vi "test Loopback_Complex_withOverflow.vi"(8 "error in":errorcluster, 11 "TestCase in":refnum<class "Single Core Complex Loopback.lvclass">) -> (0 "error out":errorcluster, 3 "TestCase out":refnum<class "Single Core Complex Loopback.lvclass">)   [LabVIEW 2020, in "Single Core Complex Loopback.lvclass"]
uses:
  Single Core Complex Loopback.lvclass
  <vilib>/addons/_JKI Toolkits/VI Tester/TestCase.llb/TestCase.lvclass
  4b06c685-66bb-4135-9ad1-d89a50a95502.vi
  <vilib>/NI VeriStand/Execution/Workspace/NI_VS Workspace ExecutionAPI.lvlib
  <vilib>/NI VeriStand/Execution/Workspace/NI VeriStand - Get Single Channel Value.vi
  <vilib>/numeric/Random Number (Range) DBL.vi
  <vilib>/NI VeriStand/Execution/Workspace/NI VeriStand - Set Single Channel Value.vi
  C:/Users/nitest/Desktop/Git 2020/niveristand-custom-device-testing-tools/VeriStandTestCase/VeriStandTestCase.lvclass
  C:/Program Files (x86)/National Instruments/LabVIEW 2020/vi.lib/addons/_JKI Toolkits/VI Tester/TestCase.llb/TestCase.lvclass
  C:/Users/nitest/Desktop/Git 2020/niveristand-ballard-arinc429-custom-device/Source/Custom Device Support/Tests/System/Single Core (P2--P3) Complex Loopback/Single Core Complex Loopback.lvclass
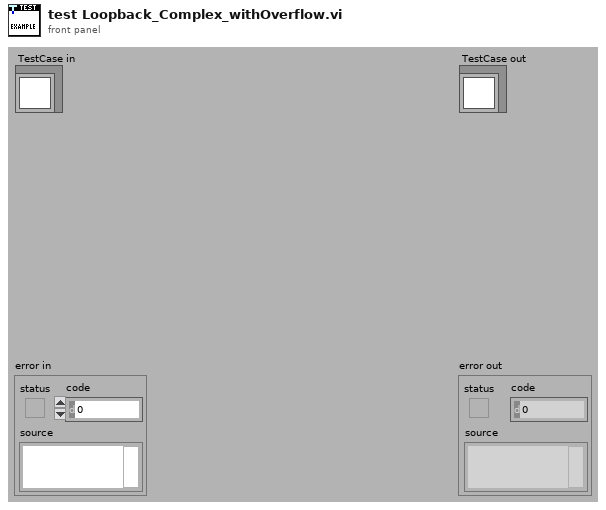
[diagram p1: front panel]
types:
  T1 = typedef "NI_VS Workspace ExecutionAPI.lvlib/WorkspaceAPI.ctl" = refnum<k24>
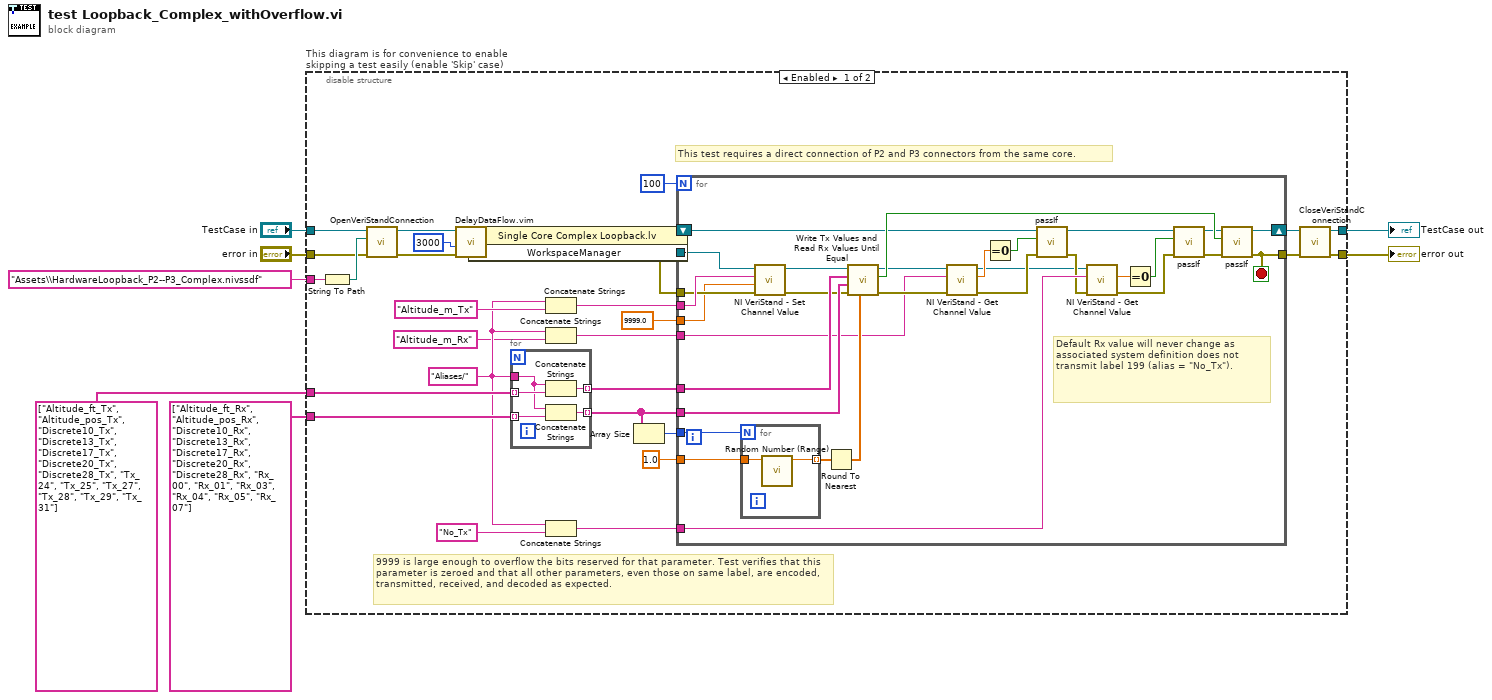
[diagram p0: block diagram]
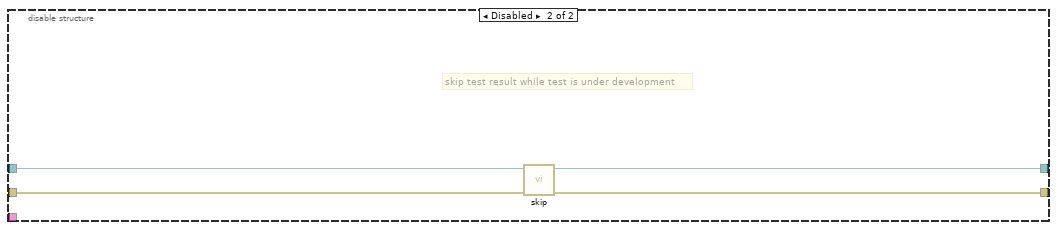
[diagram p2: hidden frame]
diagram:
  n1 = disable-structure "This diagram is for convenience to enable skipping a test easily (enable 'Skip' case)" shown="Enabled" {
    disable-tunnel: "TestCase in" -> [w32 w79]
    disable-tunnel: [w29 w77] -> w4
    disable-tunnel: [w28 w78] -> w6
    disable-tunnel: "error in" -> [w31 w76]
    disable-tunnel: "Assets\\HardwareLoopback_P2--P3_Complex.nivssdf" ("Channel") -> [w30 _]
    disable-tunnel: string[] ["Altitude_ft_Tx", "Altitude_pos_Tx", "Discrete10_Tx", "Discrete13_Tx", "Discrete17_Tx", "Discrete20_Tx", "Discrete28_Tx", "Tx_24", "Tx_25", "Tx_27", "Tx_28", "Tx_29", "Tx_31"] -> [w22 _]
    disable-tunnel: string[] ["Altitude_ft_Rx", "Altitude_pos_Rx", "Discrete10_Rx", "Discrete13_Rx", "Discrete17_Rx", "Discrete20_Rx", "Discrete28_Rx", "Rx_00", "Rx_01", "Rx_03", "Rx_04", "Rx_05", "Rx_07"] -> [w21 _]
    frame Enabled {
      w12 = "Aliases/" ("Channel")
      # "9999 is large enough to overflow the bits reserved for that parameter. Test verifies that this parameter is zeroed and that all other parameters, even those on same label, are encoded, transmitted, received, and decoded as expected."
      # "This test requires a direct connection of P2 and P3 connectors from the same core."
      n2 = String To Path(string=w30) -> (path=w33:path)
      n3 = call-dynamic "OpenVeriStandConnection.vi"("error in (no error)"=w31, "System Definition File"=w33, "VeriStand Test Case in"=w32) -> ("error out"=w35:errorcluster, "VeriStand Test Case out"=w37:refnum<class "Single Core Complex Loopback.lvclass">)  [unwired: 6 in, 1 out]
      n4 = call "DelayDataFlow.vim"("value in"=w35, "milliseconds to wait"=u32 3000) -> ("value out"=w34:errorcluster)  [unwired: 2 in, 1 out]
      n5 = property class="Single Core Complex Loopback.lv"(reference=w37, error in=w34) -> (reference out=w25:refnum<class "Single Core Complex Loopback.lvclass">, error out=w26:errorcluster, "WorkspaceManager"=w27:T1)
      n6 = for {
        tunnel: w12 -> [w40]
        tunnel: w22 -> [w42] mode=indexing
        tunnel: w21 -> [w41] mode=indexing
        tunnel: [w39] -> w20 mode=indexing
        tunnel: [w38] -> w15 mode=indexing
        n7 = Concatenate Strings(w40, w42) -> (w39:string)
        n8 = Concatenate Strings(w40, w41) -> (w38:string)
      }
      n9 = Concatenate Strings(w12, "Altitude_m_Tx" ("Channel")) -> (w10:string)
      n10 = Concatenate Strings(w12, "Altitude_m_Rx" ("Channel")) -> (w8:string)
      n11 = Concatenate Strings(w12, "No_Tx" ("Channel")) -> (w16:string)
      n12 = Array Size(array=w15) -> (size(s)=w14:i32)
      n13 = for {
        N: 100 ("x") -> [_]
        tunnel: w20 -> [w69]
        tunnel: w27 -> [w54]
        tunnel: w26 -> [w55]
        tunnel: w15 -> [w68]
        shift-right: [w73] -> w24
        shift-left: w25 -> [w48]
        tunnel: [w72] -> w23
        tunnel: 1.0 ("upper bound (100)") -> [w70]
        tunnel: w16 -> [w65]
        tunnel: w14 -> [w59]
        tunnel: w10 -> [w58]
        tunnel: 9999.0 ("Value") -> [w53]
        tunnel: w8 -> [w43]
        stop <- w72 stop-if-true
        # "Default Rx value will never change as associated system definition does not transmit label 199 (alias = \"No_Tx\")."
        n14 = for {
          N: w59 -> [_]
          tunnel: [w75] -> w71 mode=indexing
          tunnel: w70 -> [w74]
          n15 = call-poly <vilib>:"Random Number (Range).vi"("upper bound (100)"=w74) -> ("number"=w75:dbl)  [unwired: 10 in]
        }
        n16 = call-poly <vilib>:"NI VeriStand - Set Channel Value.vi"("error in (no error)"=w55, "Value"=w53, "Channel"=w58, "WorkspaceManager in"=w54) -> ("error out"=w56:errorcluster, "WorkspaceManager out"=w57:T1)  [unwired: 6 in]
        n17 = Round To Nearest(number=w71) -> (nearest integer value=w66:dbl[])
        n18 = call "Write Tx Values and Read Rx Values Until Equal.vi"("Tx values"=w66, "error in"=w56, "Rx aliases"=w68, "Tx aliases"=w69, "workspace manager in"=w57) -> ("error out"=w51:errorcluster, "values equal"=w67:bool, "workspace manager out"=w52:T1)  [unwired: 4 in]
        n19 = call-poly <vilib>:"NI VeriStand - Get Channel Value.vi"("error in (no error)"=w51, "Channel"=w43, "WorkspaceManager in"=w52) -> ("error out"=w46:errorcluster, "Value"=w50:dbl, "WorkspaceManager out"=w44:T1)  [unwired: 6 in]
        n20 = Equal To 0?(x=w50) -> (x = 0?=w49:bool)
        n21 = call-dynamic "passIf.vi"("error in (no error)"=w46, "pass"=w49, "TestCase in"=w48) -> ("error out"=w45:errorcluster, "TestCase out"=w47:refnum<class "Single Core Complex Loopback.lvclass">)  [unwired: 7 in]
        n22 = call-poly <vilib>:"NI VeriStand - Get Channel Value.vi"("error in (no error)"=w45, "Channel"=w65, "WorkspaceManager in"=w44) -> ("error out"=w63:errorcluster, "Value"=w64:dbl)  [unwired: 6 in, 1 out]
        n23 = Equal To 0?(x=w64) -> (x = 0?=w60:bool)
        n24 = call-dynamic "passIf.vi"("error in (no error)"=w63, "pass"=w60, "TestCase in"=w47) -> ("error out"=w62:errorcluster, "TestCase out"=w61:refnum<class "Single Core Complex Loopback.lvclass">)  [unwired: 7 in]
        n25 = call-dynamic "passIf.vi"("error in (no error)"=w62, "pass"=w67, "TestCase in"=w61) -> ("error out"=w72:errorcluster, "TestCase out"=w73:refnum<class "Single Core Complex Loopback.lvclass">)  [unwired: 7 in]
      }
      n26 = call-dynamic "CloseVeriStandConnection.vi"("error in (no error)"=w23, "VeriStand Test Case in"=w24) -> ("error out"=w28:errorcluster, "VeriStand Test Case out"=w29:refnum<class "Single Core Complex Loopback.lvclass">)  [unwired: 8 in]
    }
    frame Disabled {
      # "skip test result while test is under development"
      n27 = call <vilib>:"skip.vi"("error in (no error)"=w76, "TestCase in"=w79) -> ("error out"=w78:errorcluster, "TestCase in"=w77:refnum<class "Single Core Complex Loopback.lvclass">)  [unwired: 8 in]
    }
  }
  "error out" <- w6
  "TestCase out" <- w4
